vi "_Serial_Mark10-Receive data (Stand State).vi"(5 "Serial Port":refnum<visa-resource-name>="COM5") -> (1 "Motor Stop State":bool, 2 "Serial Port out":refnum<visa-resource-name>="COM5")   [LabVIEW 2015]
panel:
  out "Process Time(ms)":u32
  out "Read Buffer":string
  # "MARK10 Gauge data receive"
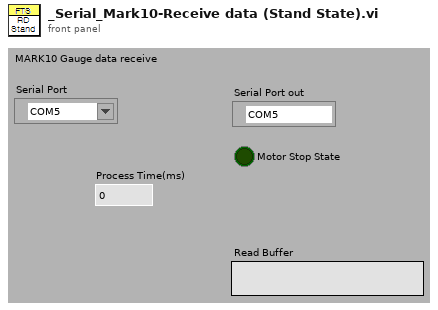
[diagram p1: front panel]
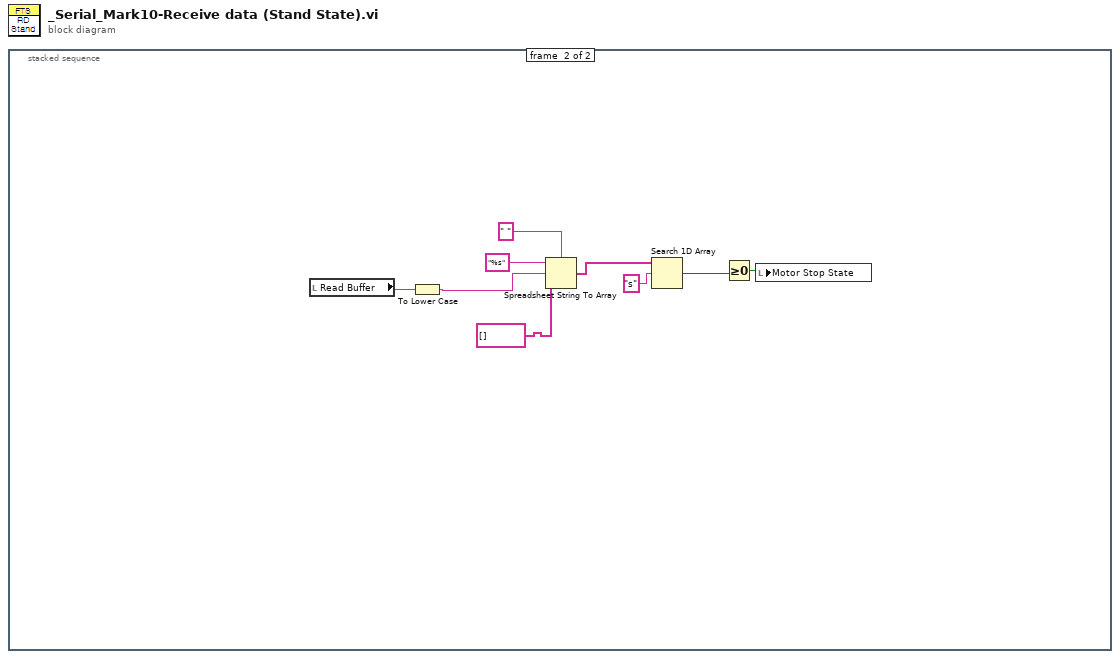
[diagram p0: block diagram]
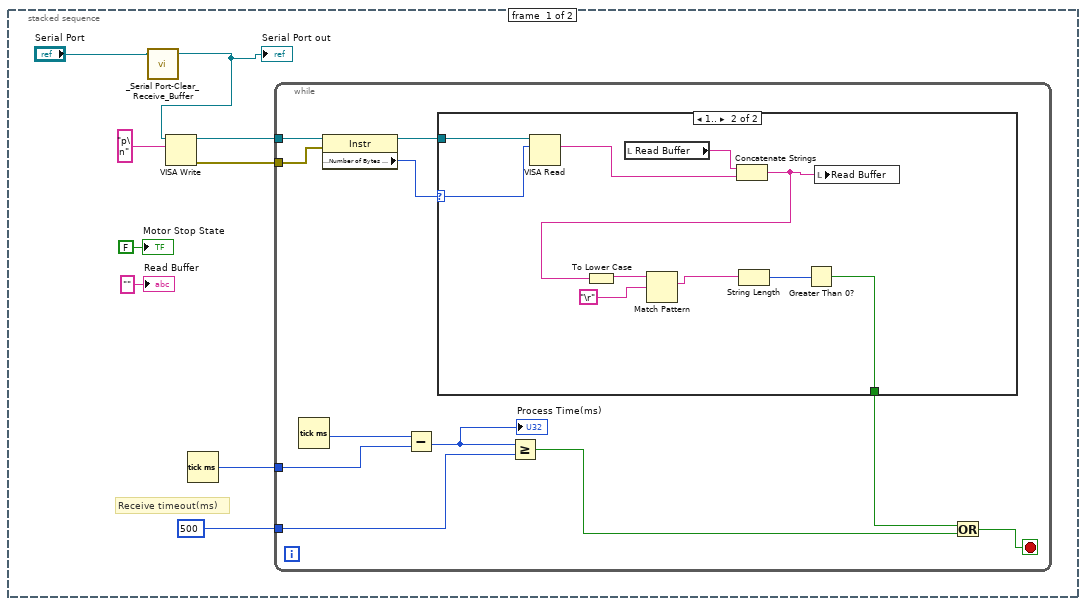
[diagram p2: hidden frame]
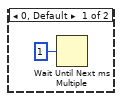
[diagram p3: hidden frame]
diagram:
  n1 = stacked-sequence {
    frame #0 {
      # "Receive timeout(ms)"
      n2 = call "_Serial Port-Clear_Receive_Buffer.vi"("Serial Port"="Serial Port") -> ("Serial Port out"=w1:refnum<visa-resource-name>)  [unwired: 3 in, 1 out]
      "Serial Port out" <- w1
      n3 = VISA Write(VISA resource name=w1, write buffer="p\n") -> (VISA resource name out=w7:refnum<visa-resource-name>, error out=w6:errorcluster)  [unwired: 1 in, 1 out]
      n4 = Tick Count (ms)() -> (millisecond timer value=w5:u32)
      n5 = while {
        tunnel: w7 -> [w19]
        tunnel: w6 -> [w18]
        tunnel: w5 -> [w15]
        tunnel: 500 -> [w13]
        stop <- w11 stop-if-true
        n6 = Tick Count (ms)() -> (millisecond timer value=w16:u32)
        n7 = property class="Instr"(reference=w19, error in=w18) -> (reference out=w20:refnum<visa-resource-name>, "Serial Settings:Number of Bytes at Serial Port"=w17:u32)  [unwired: 1 out]
        n8 = Subtract(x=w16, y=w15) -> (x-y=w14:u32)
        "Process Time(ms)" <- w14
        n9 = case shown="1.." w17 {
          selector: w17 -> [_ w24]
          tunnel: w20 -> [_ w31]
          tunnel: [_ w25] -> w10
          frame 0, Default {
            n10 = Wait Until Next ms Multiple(millisecond multiple=u32 1 ("ms 배수")) -> ()  [unwired: 1 out]
          }
          frame 1.. {
            n11 = VISA Read(VISA resource name=w31, byte count=w24) -> (read buffer=w29:string)  [unwired: 1 in, 3 out]
            n12 = local read "Read Buffer"() -> (w30:string)
            n13 = Concatenate Strings(w30, w29) -> (w28:string)
            n14 = To Lower Case(string=w28) -> (all lower case string=w27:string)
            n15 = Match Pattern(string=w27, regular expression="\r") -> (match substring=w23:string)  [unwired: 1 in, 3 out]
            n16 = String Length(string=w23) -> (length=w26:i32)
            n17 = Greater Than 0?(x=w26) -> (x > 0?=w25:bool)
            n18 = local write "Read Buffer"(w28) -> ()
          }
        }
        n19 = Greater Or Equal?(x=w14, y=w13) -> (x >= y?=w12:bool)
        n20 = Or(x=w10, y=w12) -> (x .or. y?=w11:bool)
      }
      "Motor Stop State" <- FALSE ("수신 정상")
      "Read Buffer" <- "" ("버퍼 읽기")
    }
    frame #1 {
      n21 = local read "Read Buffer"() -> (w40:string)
      n22 = To Lower Case(string=w40) -> (all lower case string=w37:string)
      n23 = Spreadsheet String To Array(delimiter (Tab)=" " ("구분 문자(탭)"), format string="%s" ("포맷 문자열"), spreadsheet string=w37, array type (2D Dbl)=string[] [] ("배열 타입(2D Dbl)")) -> (array=w35:string[])
      n24 = Search 1D Array(1D array=w35, element="s" ("원소")) -> (index of element=w32:i32)  [unwired: 1 in]
      n25 = Greater Or Equal To 0?(x=w32) -> (x >= 0?=w33:bool)
      n26 = local write "Motor Stop State"(w33) -> ()
    }
  }
